vi "ESP8266.vi"() -> ()   [LabVIEW 2023]
uses:
  <vilib>/Instr/_visa.llb/VISA Configure Serial Port (Instr).vi
panel:
  out "已停车位数量":dbl
  out "剩余车位数量":dbl
  out "布尔 17":bool caption="布尔"
  out "布尔 16":bool caption="布尔"
  out "布尔 15":bool caption="布尔"
  out "布尔 14":bool caption="布尔"
  out "布尔 13":bool caption="布尔"
  out "布尔 12":bool caption="布尔"
  out "布尔 11":bool caption="布尔"
  out "布尔 10":bool caption="布尔"
  out "布尔 9":bool caption="布尔"
  out "布尔 8":bool caption="布尔"
  out "布尔 7":bool caption="布尔"
  out "布尔":bool
  out "布尔 6":bool caption="布尔"
  out "布尔 5":bool caption="布尔"
  out "布尔 4":bool caption="布尔"
  out "布尔 3":bool caption="布尔"
  out "布尔 2":bool caption="布尔"
  out "布尔":bool
  out "读取缓冲区":string
  out "错误输出":errorcluster
  out "返回数":u32
  # "停车位检测系统"
  # "车位即时显示图"
  # "系统状态显示区"
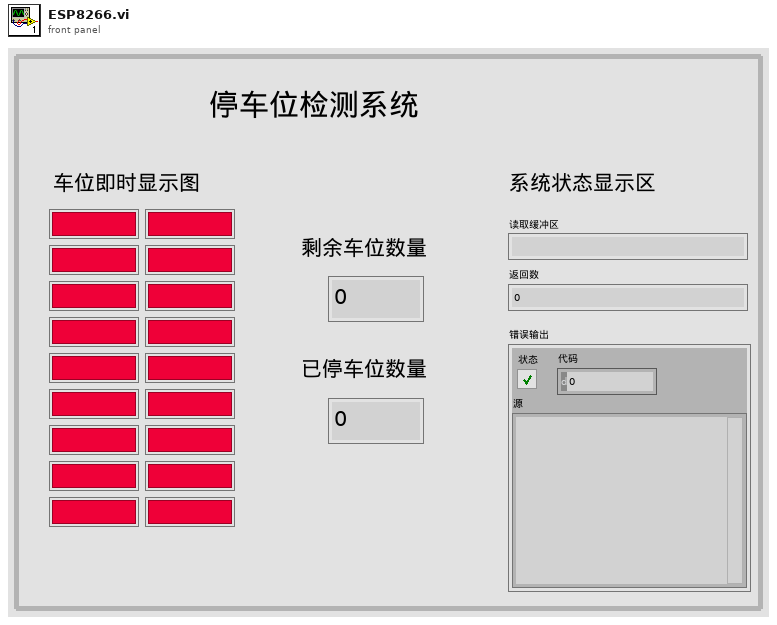
[diagram p1: front panel]
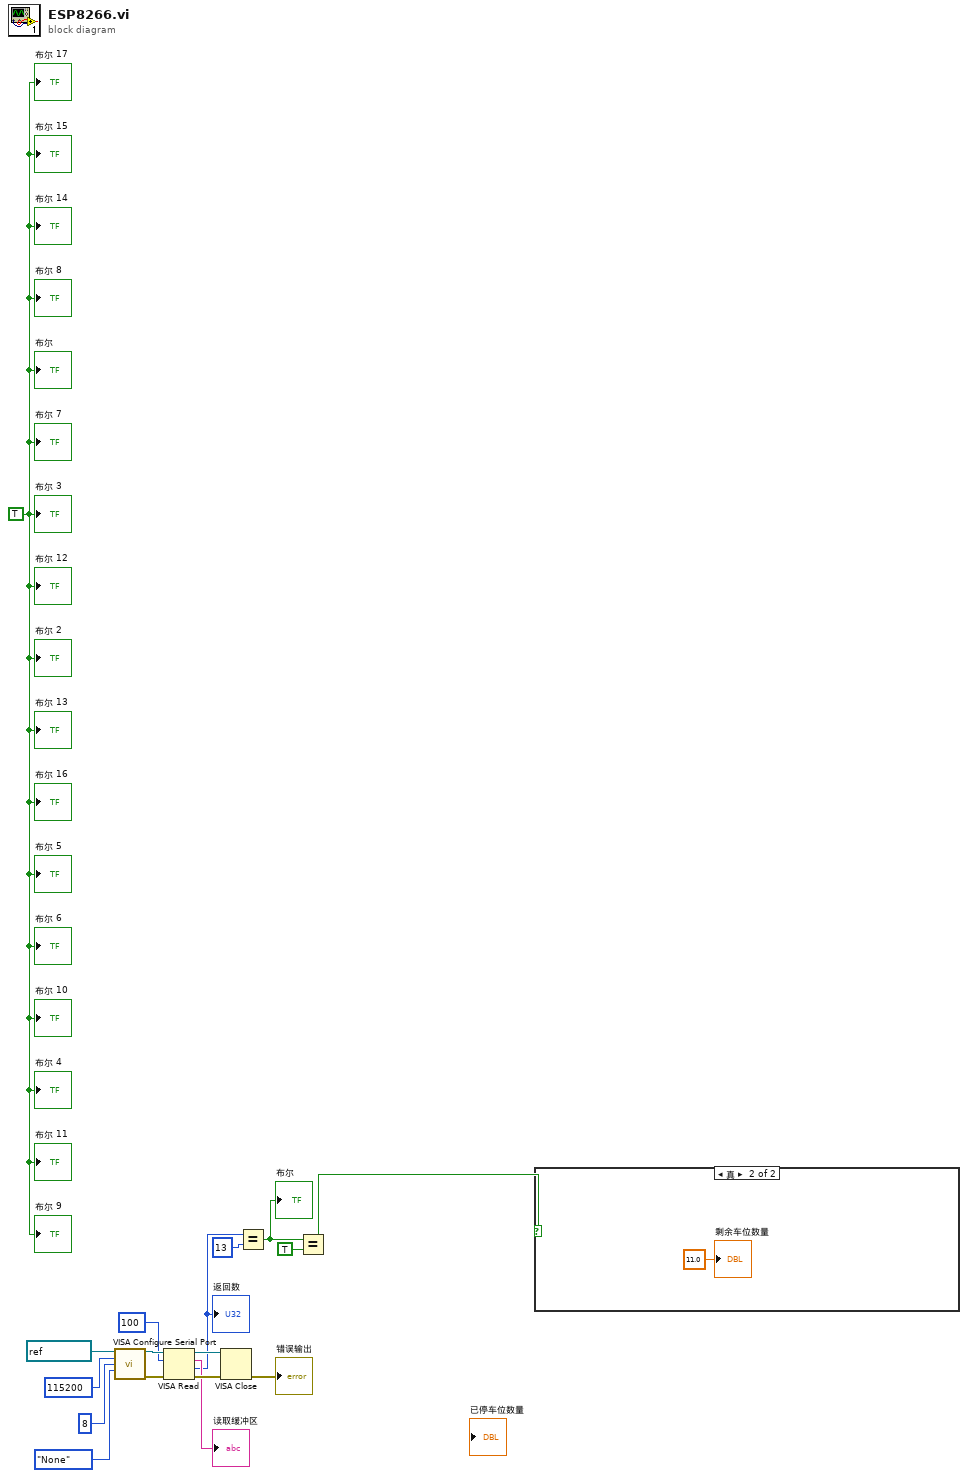
[diagram p0: block diagram]
diagram:
  w2 = TRUE ("布尔 6")
  n1 = call-poly "VISA Configure Serial Port"("VISA resource name"=refnum<visa-resource-name> "COM8", "baud rate (9600)"=u32 115200, "data bits (8)"=u16 8, "parity (0:none)"=enum16{"None", "Odd", "Even", "Mark", "Space"}."None") -> ("VISA resource name out"=w16:refnum<visa-resource-name>, "error out"=w14:errorcluster)  [unwired: 10 in]
  n2 = VISA Read(VISA resource name=w16, byte count=u32 100 ("字节总数"), error in (no error)=w14) -> (VISA resource name out=w12:refnum<visa-resource-name>, read buffer=→"读取缓冲区":string, return count=w6:u32, error out=w9:errorcluster)
  "返回数" <- w6
  n3 = VISA Close(VISA resource name=w12, error in (no error)=w9) -> (error out=→"错误输出":errorcluster)
  n4 = Equal?(x=w6, y=u32 13) -> (x = y?=w4:bool)
  "布尔" <- w4
  n5 = Equal?(x=w4, y=TRUE) -> (x = y?=w1:bool)
  n6 = case shown="真" w1 {
    frame False {
    }
    frame True {
      "剩余车位数量" <- 11.0 ("剩余车位数量")
    }
  }
  "布尔 2" <- w2
  "布尔 3" <- w2
  "布尔 4" <- w2
  "布尔 5" <- w2
  "布尔 6" <- w2
  "布尔" <- w2
  "布尔 7" <- w2
  "布尔 8" <- w2
  "布尔 9" <- w2
  "布尔 10" <- w2
  "布尔 11" <- w2
  "布尔 12" <- w2
  "布尔 13" <- w2
  "布尔 14" <- w2
  "布尔 15" <- w2
  "布尔 16" <- w2
  "布尔 17" <- w2
